vi "Get - Vector - Strings.vi"(5 "use temporary file?":bool, 7 "data type of variable":string[](array[string]), 8 "error in":errorcluster, 10 "variable name":string, 11 "pipe in":T1) -> (0 "error out":errorcluster, 2 "value":string[](array[string]), 3 "pipe out":T1)   [LabVIEW 2013, in "GOLPI library.lvlib"]
uses:
  GOLPI library.lvlib
  LV Process.lvlibp/Pipe Handle.ctl
  Custom Error Codes Enum Type Def.vi
  LV Process.lvlibp
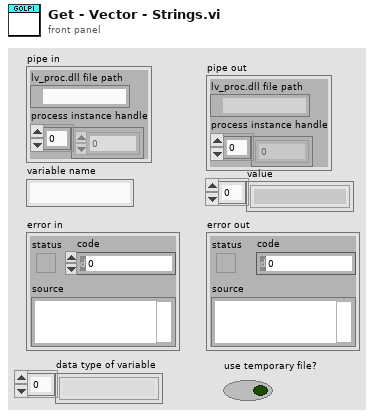
[diagram p1: front panel]
types:
  T1 = typedef "LV Process.lvlibp/Pipe Handle.ctl" = cluster{"lv_proc.dll file path":path, "process instance handle":u32[]}
  T2 = typedef "GOLPI library.lvlib/Custom Error Codes Enum Type Def.vi" = enum16{"no error", "00 working directory PAR1 missing", "01 octave binary PAR1 missing", "02 octave report error PAR1", "03 empty output last cmd PAR1", "04 missing temporary file PAR1", "10 var PAR1 not string", "11 var PAR1 not num, scal, ~compl", "12 var PAR1 not num, scal, compl", "13 var PAR1 not num, vect, ~compl", "14 var PAR1 not num, vect, compl", "15 var PAR1 not num, mat, ~compl", "16 var PAR1 not num, mat, ~compl", "99 not finished"}
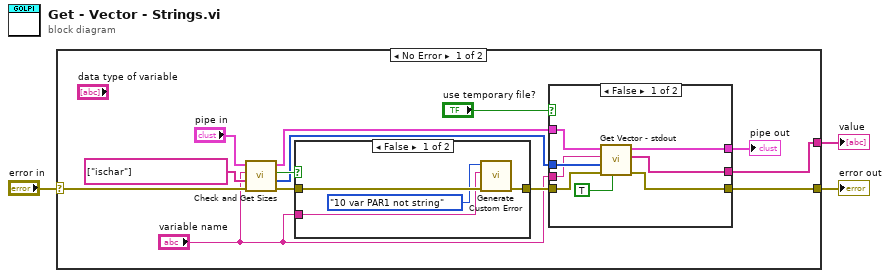
[diagram p0: block diagram]
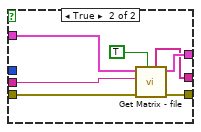
[diagram p2: hidden frame]
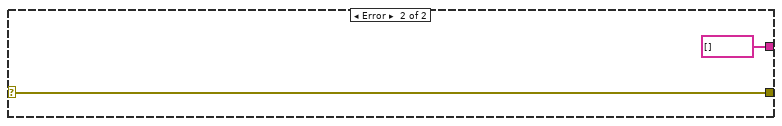
[diagram p4: hidden frame]
diagram:
  n1 = case shown="No Error" "error in" {
    selector: "error in" -> [w13 w38]
    tunnel: [w7 w38] -> w3
    tunnel: [w16 string[] [] ("vector")] -> w1
    frame No Error {
      n2 = call "Check and Get Sizes.vi"("error in (no error)"=w13, "test commands"=string[] ["ischar"], "variable name"="variable name", "pipe in"="pipe in") -> ("error out"=w12:errorcluster, "octave sizes"=w9:i32[], "all tests OK?"=w14:bool, "pipe out"=w10:T1)  [unwired: 4 in]
      n3 = case shown="False" w14 {
        tunnel: w12 -> [w35 w36]
        tunnel: [w32 w36] -> w8
        tunnel: "variable name" -> [w33 _]
        frame False {
          n4 = call "Generate Custom Error.vi"("error in"=w35, "PAR1"=w33, "GOLPI error"=Custom_Error_Codes_Enum_Type_Def.vi."10 var PAR1 not string" ("Enum")) -> ("error out"=w32:errorcluster)  [unwired: 8 in]
        }
        frame True {
        }
      }
      n5 = case shown="False" "use temporary file?" {
        tunnel: [w17 w26] -> w16
        tunnel: w10 -> [w24 w29]
        tunnel: w9 -> [w23 _]
        tunnel: w8 -> [w22 w31]
        tunnel: [w21 w30] -> w7
        tunnel: "variable name" -> [w19 w27]
        tunnel: [w18 w28] -> w4
        frame False {
          n6 = call "Get Vector - stdout.vi"("no transpose\nfor reading"=TRUE ("no transpose\nwhen reading"), "error in (no error)"=w22, "octave vector sizes"=w23, "variable name"=w19, "pipe in"=w24) -> ("error out"=w21:errorcluster, "vector"=w17:string[], "pipe out"=w18:T1)  [unwired: 3 in, 1 out]
        }
        frame True {
          n7 = call "Get Matrix - file.vi"("is string"=TRUE, "error in (no error)"=w31, "variable name"=w27, "pipe in"=w29) -> ("error out"=w30:errorcluster, "pipe out"=w28:T1, "string array"=w26:string[])  [unwired: 3 in, 2 out]
        }
      }
      "pipe out" <- w4
    }
    frame Error {
    }
  }
  "value" <- w1
  "error out" <- w3
